vi "MoveElevatorUp.vi"(8 "error in (no error)":errorcluster) -> (0 "error out":errorcluster)   [LabVIEW 2017, in "Thermal Shock.lvlib"]
uses:
  Thermal Shock.lvlib
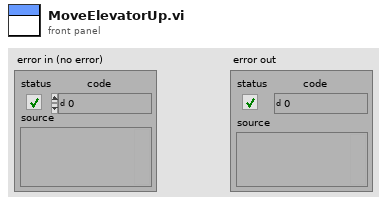
[diagram p1: front panel]
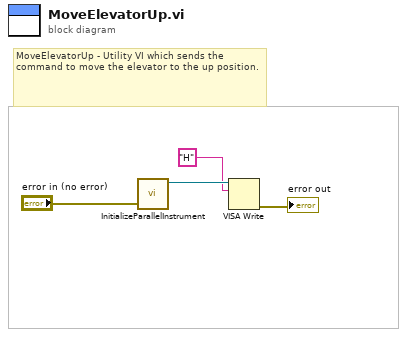
[diagram p0: block diagram]
diagram:
  # "MoveElevatorUp - Utility VI which sends the command to move the elevator to the up position."
  n1 = call "InitializeParallelInstrument.vi"("error in (no error)"="error in (no error)") -> ("Parallel Instrument OUT"=w4:refnum<visa-resource-name>)  [unwired: 9 in, 1 out]
  n2 = VISA Write(VISA resource name=w4, write buffer="H") -> (error out=→"error out":errorcluster)  [unwired: 1 in, 2 out]
